vi "LinearSystemLoop_Predict.vi"(6 "dT_Seconds":dbl, 11 "input inear System Loop":T1) -> (0 "Error":bool, 3 "out Linear System Loop":T1)   [LabVIEW 2019, in "Trajectory_Library.lvlib"]
doc: "Sets new controller output, projects model forward, and runs observer prediction.\n \nAfter calling this, the user should send the elements of u to the actuators.\n \nInputs:\n - LinearSystemLoop -- system data cluster\n - dtSeconds -- Timestep for model update.\n\nOutputs:\n - outLinearSystemLoop -- updated system data cluster\n - error -- If TRUE, an error occured."
uses:
  Trajectory_Library.lvlib
  <vilib>/Analysis/Matrix/NI_Matrix.lvlib
  <vilib>/Analysis/Matrix/Numeric/Add/Add - RM,RM.vi
  TypeDef/LINEAR_SYSTEM.ctl
  <vilib>/Analysis/Matrix/Datatypes/RealMatrix.ctl
  TypeDef/LINEAR_QUADRATIC_REGULATOR.ctl
  TypeDef/LINEAR_PLANT_INV_FF.ctl
  TypeDef/KALMAN_FILTER.ctl
  TypeDef/LINEAR_SYSTEM_LOOP.ctl
panel:
  # "<States,1>"
  # "<FUTURE --- CLAMP TYPE -- For now\nuse Normalize>"
  # "Steady State Gain  \n<States,Outputs>"
  # "State Estimate <Statess,1>"
  # "<States,States>"
  # "<States,Inputs>"
  # "<Outputs,States>"
  # "<Outputs,Inputs>"
  # "<States,1>"
  # "<Inputs,1>"
  # "<States,Inputs>"
  # "<States,States>"
  # "Ref State <States,1>"
  # "Comp and capped \noutput <Inputs,1>"
  # "Controller gain\n<Inputs,States>"
  # "<States,1>"
  # "<FUTURE --- CLAMP TYPE -- For now\nuse Normalize>"
  # "Steady State Gain  \n<States,Outputs>"
  # "State Estimate <Statess,1>"
  # "<States,States>"
  # "<States,Inputs>"
  # "<Outputs,States>"
  # "<Outputs,Inputs>"
  # "<States,1>"
  # "<Inputs,1>"
  # "<States,Inputs>"
  # "<States,States>"
  # "Ref State <States,1>"
  # "Comp and capped \noutput <Inputs,1>"
  # "Controller gain\n<Inputs,States>"
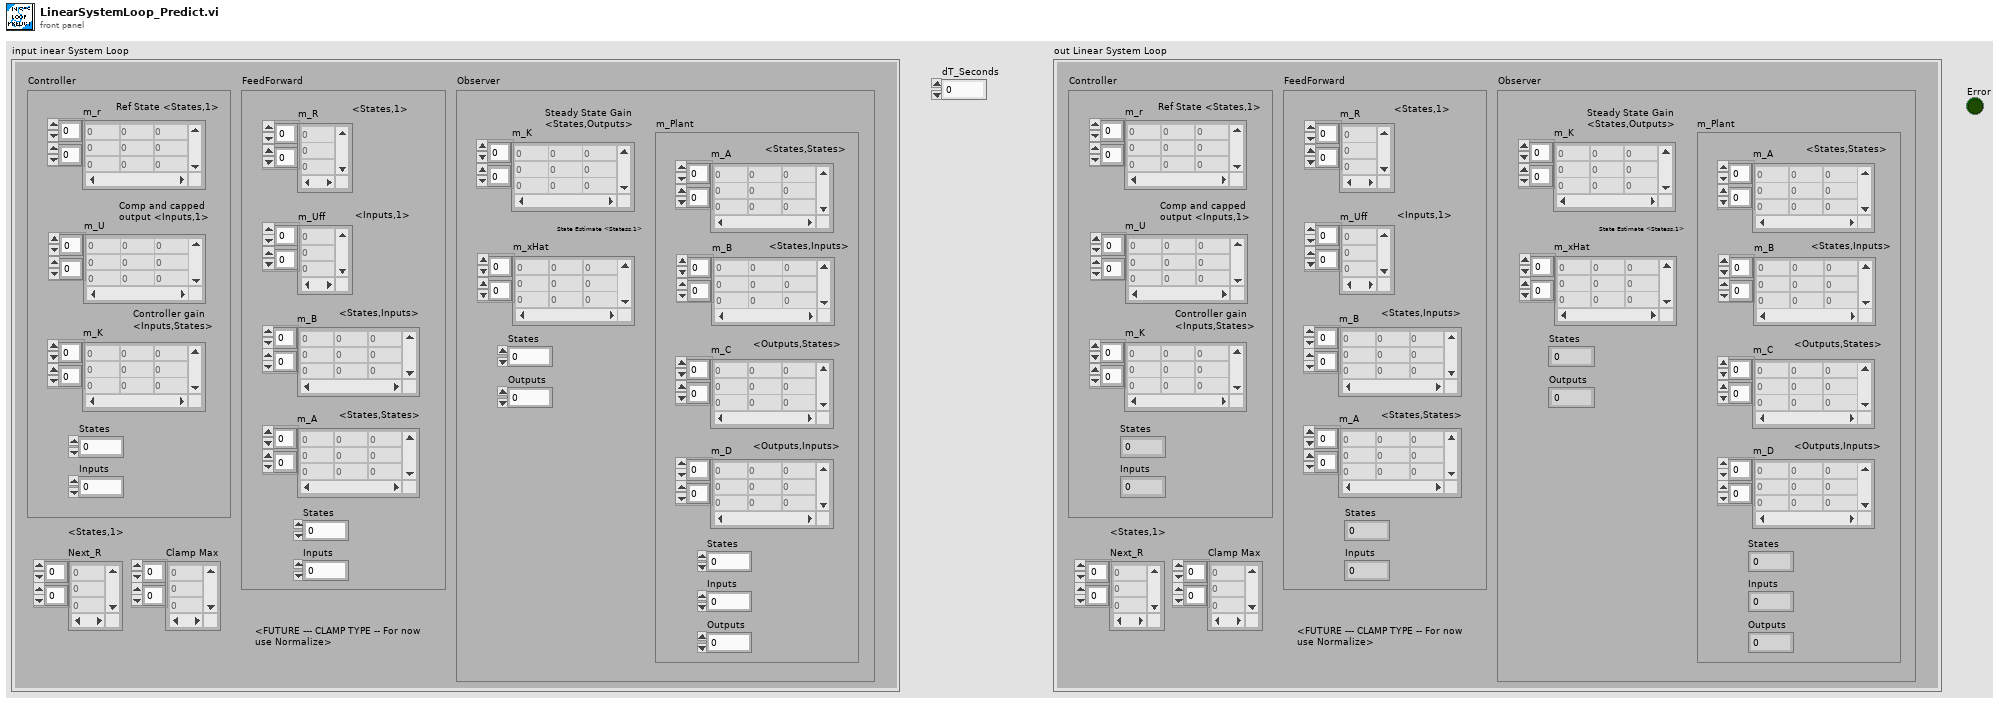
[diagram p1: front panel]
types:
  T1 = typedef "Trajectory_Library.lvlib/LINEAR_SYSTEM_LOOP.ctl" = cluster{"Controller":T2, "FeedForward":T4, "Observer":T5, "Next_R":T3, "Clamp Max":T3}
  T2 = typedef "Trajectory_Library.lvlib/LINEAR_QUADRATIC_REGULATOR.ctl" = cluster{"m_r":T3, "m_U":T3, "m_K":T3, "States":i32, "Inputs":i32}
  T3 = typedef "NI_Matrix.lvlib/RealMatrix.ctl" = dbl[][]
  T4 = typedef "Trajectory_Library.lvlib/LINEAR_PLANT_INV_FF.ctl" = cluster{"m_R":T3, "m_Uff":T3, "m_B":T3, "m_A":T3, "States":i32, "Inputs":i32}
  T5 = typedef "Trajectory_Library.lvlib/KALMAN_FILTER.ctl" = cluster{"m_K":T3, "m_xHat":T3, "States":i32, "Outputs":i32, "m_Plant":T6}
  T6 = typedef "Trajectory_Library.lvlib/LINEAR_SYSTEM.ctl" = cluster{"m_A":T3, "m_B":T3, "m_C":T3, "m_D":T3, "States":i32, "Inputs":i32, "Outputs":i32}
  T7 = typedef "WPILib_Math.lvlib/LINEAR_QUADRATIC_REGULATOR.ctl" = cluster{"m_r":T3, "m_U":T3, "m_K":T3, "States":i32, "Inputs":i32}
  T8 = typedef "WPILib_Math.lvlib/LINEAR_PLANT_INV_FF.ctl" = cluster{"m_R":T3, "m_Uff":T3, "m_B":T3, "m_A":T3, "States":i32, "Inputs":i32}
  T9 = typedef "WPILib_Math.lvlib/KALMAN_FILTER.ctl" = cluster{"m_K":T3, "m_xHat":T3, "States":i32, "Outputs":i32, "m_Plant":T10}
  T10 = typedef "WPILib_Math.lvlib/LINEAR_SYSTEM.ctl" = cluster{"m_A":T3, "m_B":T3, "m_C":T3, "m_D":T3, "States":i32, "Inputs":i32, "Outputs":i32}
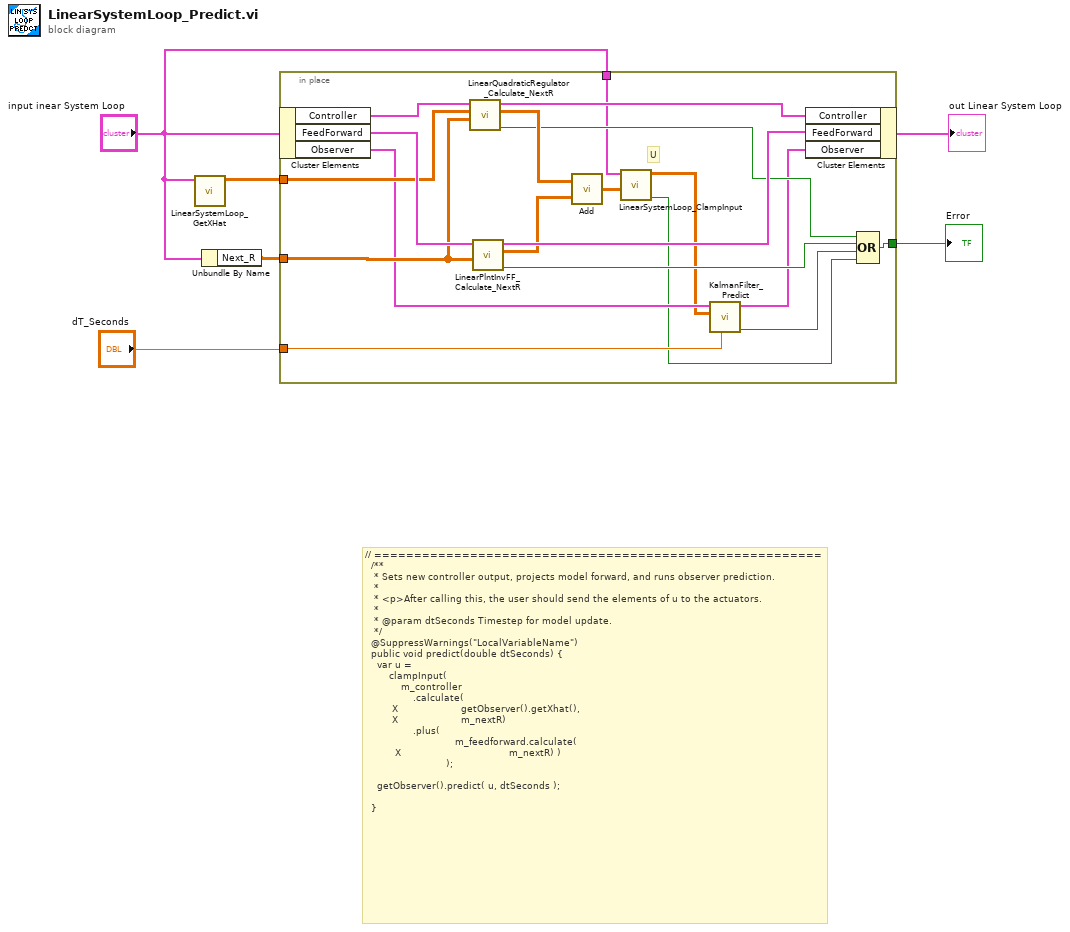
[diagram p0: block diagram]
diagram:
  # "// ========================================================\n  /**\n   * Sets new controller output, projects model forward, and runs observer prediction.\n   *\n   * <p>After calling this, the user should send the elements of u to the actuators.\n   *\n   * @param dtSeconds Timestep for model update.\n   */\n  @SuppressWarnings(\"LocalVariableName\")\n  public void predict(double dtSeconds) {\n    var u =\n        clampInput(    \n            m_controller\n                .calculate(\n         X                     getObserver().getXhat(), \n         X                     m_nextR)\n                .plus(\n                              m_feedforward.calculate(\n          X                                    m_nextR) )\n                           );\n\n    getObserver().predict( u, dtSeconds );\n\n  }"
  n1 = call "LinearSystemLoop_GetXHat.vi"("input inear System Loop"="input inear System Loop") -> ("XHat"=w2:T3)  [unwired: 10 in]
  n2 = Unbundle By Name("input inear System Loop") -> ("Next_R"=w5:T3)
  n3 = in-place {
    in-place-border: w5 -> [w17]
    in-place-border: [w21] -> w4
    in-place-border: w2 -> [w18]
    in-place-border: "dT_Seconds" -> [w12]
    in-place-border: "input inear System Loop" -> [w8]
    # "U"
    n4 = in-place-cluster #1("input inear System Loop") -> ("Controller"=w20:T2, "FeedForward"=w25:T4, "Observer"=w14:T5)
    n5 = call "LinearQuadraticRegulator_Calculate_NextR.vi"("NextR"=w17, "X"=w18, "in LinearQuadraticRegulator"=w20) -> ("Error"=w15:bool, "U"=w16:T3, "out LinearQuadraticRegulator"=w19:T7)  [unwired: 6 in]
    n6 = call "LinearPlntInvFF_Calculate_NextR.vi"("NextR"=w17, "Input Linear Plant Inv FF"=w25) -> ("Error"=w22:bool, "Uff"=w23:T3, "Output Linear Plant Inv FF"=w24:T8)  [unwired: 7 in]
    n7 = call-poly <vilib>:"Add.vi"("Real Matrix B"=w23, "Real Matrix A"=w16) -> ("A + B"=w10:T3)
    n8 = call "LinearSystemLoop_ClampInput.vi"("UnclampedU"=w10, "input inear System Loop"=w8) -> ("Size Coerced"=w7:bool, "U"=w9:T3)  [unwired: 8 in]
    n9 = call "KalmanFilter_Predict.vi"("dT_Seconds"=w12, "U"=w9, "in KalmanFilter"=w14) -> ("Error"=w11:bool, "out KalmanFilter"=w13:T9)  [unwired: 7 in]
    n10 = in-place-cluster #1("Controller"=w19, "FeedForward"=w24, "Observer"=w13) -> (→"out Linear System Loop":T1)
    n11 = Compound Arithmetic op=OR(w15, w22, w11, w7) -> (w21:bool)
  }
  "Error" <- w4
